vi "Initialize Actor.vi"(7 "Host Name":string, 8 "error in (no error)":errorcluster, 9 "Actor Name":string, 10 "Message Broker Interface":refnum<class "Message Broker Interface.lvclass">, 11 "Car Wash Console in":refnum<class "Car Wash Display.lvclass">) -> (0 "error out":errorcluster, 3 "Car Wash Console out":refnum<class "Car Wash Display.lvclass">)   [LabVIEW 2016, in "CLD Exam - Car Wash.lvlib" / "Car Wash Display.lvclass"]
doc: "--\nCopyright © 2017 Composed SystemsI All rights reserved.\n\nAuthor: Jon McBee <jon.mcbee@composed.io>\n\nThis library is provided \"AS IS\" ,WITHOUT WARRANTIES OR\nCONDITIONS OF ANY KIND, either express or implied.\n\nComposed Systems -- composed.io\n\nStream 0.0.1.1\nJon McBee - Composed Systems\nCopyright (c) 2017, Composed Systems"
uses:
  Car Wash Display.lvclass
  Mediator/Classes/Message Broker Interface/Message Broker Interface.lvclass
  Car Wash Display.lvclass/Car Wash Display.ctl
  Mediator/Classes/Message Transport Event/Message Transport Event.lvclass
  D:/Repos/Stream/software/Mediator/Classes/Message Transport Interface/Message Transport Interface.lvclass
  Mediator/Classes/Mediated Synchronous Actor/Mediated Synchronous Actor.lvclass
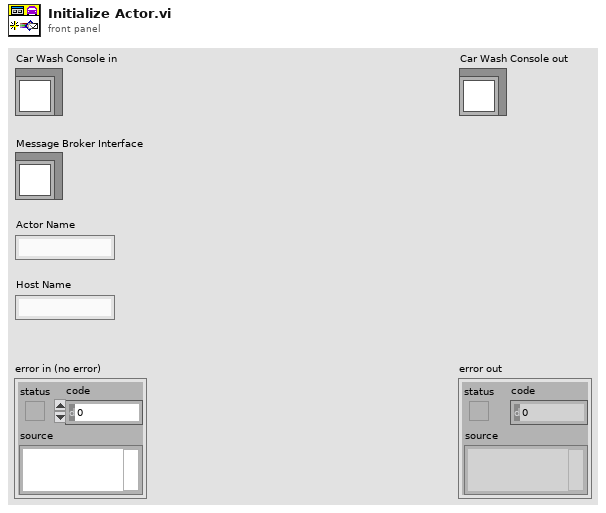
[diagram p1: front panel]
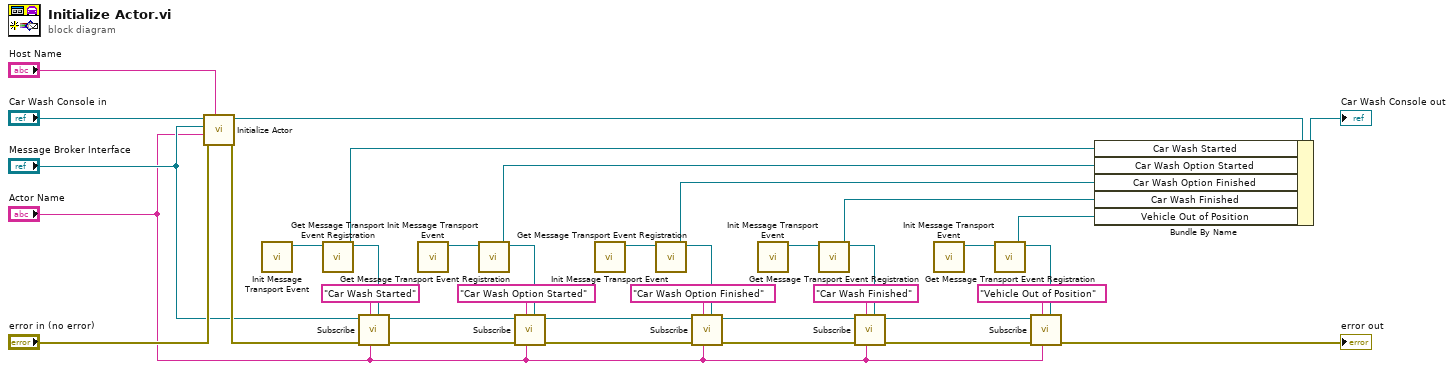
[diagram p0: block diagram]
diagram:
  n1 = call-parent "Initialize Actor.vi"("Host Name"="Host Name", "error in (no error)"="error in (no error)", "Actor Name"="Actor Name", "Message Broker Interface"="Message Broker Interface", "Mediated Synchronous Actor in"="Car Wash Console in") -> ("error out"=w29:errorcluster, "Mediated Synchronous Actor out"=w34:refnum<class "Car Wash Display.lvclass">)  [unwired: 5 in]
  n2 = call "Init Message Transport Event.vi"() -> ("Message Transport Event out"=w32:refnum<class "Message Transport Event.lvclass">)  [unwired: 10 in, 1 out]
  n3 = call "Get Message Transport Event Registration.vi"("Message Transport Event in"=w32) -> ("Event Registration Refnum"=w27:refnum<event-registration>, "Message Transport Event out"=w30:refnum<class "Message Transport Event.lvclass">)  [unwired: 7 in, 2 out]
  n4 = call-dynamic "Subscribe.vi"("Message Transport Interface"=w30, "Subscriber Name"="Actor Name", "Topic Name"="Car Wash Started", "error in (no error)"=w29, "Message Broker Interface in"="Message Broker Interface") -> ("error out"=w17:errorcluster, "Message Broker Interface out"=w23:refnum<class "Message Broker Interface.lvclass">)  [unwired: 4 in, 1 out]
  n5 = call "Init Message Transport Event.vi"() -> ("Message Transport Event out"=w24:refnum<class "Message Transport Event.lvclass">)  [unwired: 10 in, 1 out]
  n6 = call "Get Message Transport Event Registration.vi"("Message Transport Event in"=w24) -> ("Event Registration Refnum"=w22:refnum<event-registration>, "Message Transport Event out"=w26:refnum<class "Message Transport Event.lvclass">)  [unwired: 7 in, 2 out]
  n7 = call-dynamic "Subscribe.vi"("Message Transport Interface"=w26, "Subscriber Name"="Actor Name", "Topic Name"="Car Wash Option Started", "error in (no error)"=w17, "Message Broker Interface in"=w23) -> ("error out"=w16:errorcluster, "Message Broker Interface out"=w18:refnum<class "Message Broker Interface.lvclass">)  [unwired: 4 in, 1 out]
  n8 = call "Init Message Transport Event.vi"() -> ("Message Transport Event out"=w21:refnum<class "Message Transport Event.lvclass">)  [unwired: 10 in, 1 out]
  n9 = call "Get Message Transport Event Registration.vi"("Message Transport Event in"=w21) -> ("Event Registration Refnum"=w15:refnum<event-registration>, "Message Transport Event out"=w19:refnum<class "Message Transport Event.lvclass">)  [unwired: 7 in, 2 out]
  n10 = call-dynamic "Subscribe.vi"("Message Transport Interface"=w19, "Subscriber Name"="Actor Name", "Topic Name"="Car Wash Option Finished", "error in (no error)"=w16, "Message Broker Interface in"=w18) -> ("error out"=w11:errorcluster, "Message Broker Interface out"=w10:refnum<class "Message Broker Interface.lvclass">)  [unwired: 4 in, 1 out]
  n11 = call "Init Message Transport Event.vi"() -> ("Message Transport Event out"=w12:refnum<class "Message Transport Event.lvclass">)  [unwired: 10 in, 1 out]
  n12 = call "Get Message Transport Event Registration.vi"("Message Transport Event in"=w12) -> ("Event Registration Refnum"=w9:refnum<event-registration>, "Message Transport Event out"=w14:refnum<class "Message Transport Event.lvclass">)  [unwired: 7 in, 2 out]
  n13 = call-dynamic "Subscribe.vi"("Message Transport Interface"=w14, "Subscriber Name"="Actor Name", "Topic Name"="Car Wash Finished", "error in (no error)"=w11, "Message Broker Interface in"=w10) -> ("error out"=w3:errorcluster, "Message Broker Interface out"=w5:refnum<class "Message Broker Interface.lvclass">)  [unwired: 4 in, 1 out]
  n14 = call "Init Message Transport Event.vi"() -> ("Message Transport Event out"=w8:refnum<class "Message Transport Event.lvclass">)  [unwired: 10 in, 1 out]
  n15 = call "Get Message Transport Event Registration.vi"("Message Transport Event in"=w8) -> ("Event Registration Refnum"=w1:refnum<event-registration>, "Message Transport Event out"=w6:refnum<class "Message Transport Event.lvclass">)  [unwired: 7 in, 2 out]
  n16 = call-dynamic "Subscribe.vi"("Message Transport Interface"=w6, "Subscriber Name"="Actor Name", "Topic Name"="Vehicle Out of Position", "error in (no error)"=w3, "Message Broker Interface in"=w5) -> ("error out"=→"error out":errorcluster)  [unwired: 4 in, 2 out]
  n17 = Bundle By Name(cluster=w34, "Car Wash Started"=w27, "Car Wash Option Started"=w22, "Car Wash Option Finished"=w15, "Car Wash Finished"=w9, "Vehicle Out of Position"=w1) -> (→"Car Wash Console out":refnum<class "Car Wash Display.lvclass">)
